vi "reportTaskState.vi"(7 "TaskRef":refnum<vi>, 8 "error in (no error)":errorcluster, 10 "Request":string, 11 "pdbm_taskroute_feedback_event":refnum<user-event>) -> (0 "error out":errorcluster, 3 "pdbm_taskroute_feedback_event out":refnum<user-event>, 5 "TaskRef out":refnum<vi>)   [LabVIEW 2015, in "pdbm_tasks.lvlib"]
uses:
  pdbm_tasks.lvlib
  pdbm_test_route/UsrDefine/TaskFeedbackCmd.ctl
  UsrDefine/TaskRequest.ctl
  pdbm_test_route/pdbm_task_route.lvlib
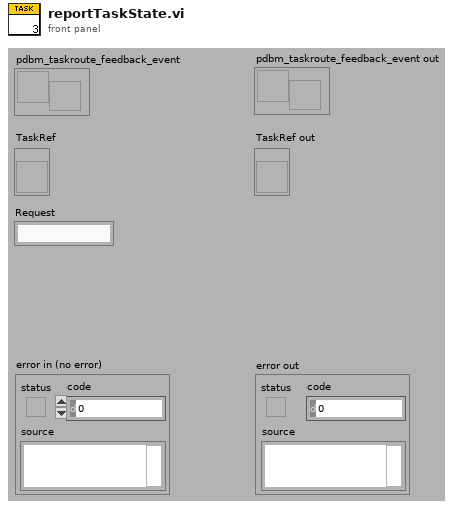
[diagram p1: front panel]
types:
  T1 = typedef "pdbm_tasks.lvlib/TaskRequest.ctl" = cluster{"Command":string, "Variant":variant}
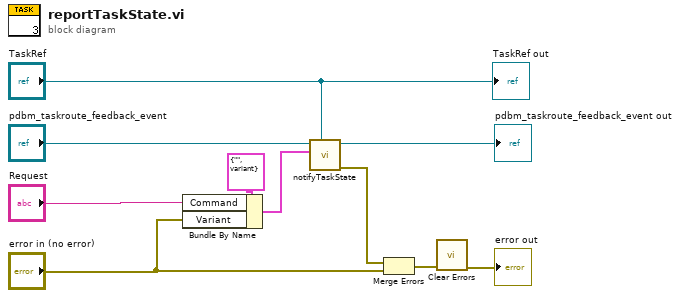
[diagram p0: block diagram]
diagram:
  n1 = Bundle By Name(cluster=T1 {"Command"="", "Variant"=variant} ("TaskRequest"), "Command"="Request", "Variant"="error in (no error)") -> (w7:T1)
  n2 = call "notifyTaskState.vi"("TaskRef"="TaskRef", "TaskRequest"=w7, "pdbm_taskroute_feedback_event"="pdbm_taskroute_feedback_event") -> ("error IO"=w3:errorcluster, "pdbm_taskroute_feedback_event out"=→"pdbm_taskroute_feedback_event out":refnum<user-event>)  [unwired: 7 in]
  n3 = Merge Errors(w3, "error in (no error)") -> (w2:errorcluster)
  n4 = call <vilib>:"Clear Errors.vi"("error in (no error)"=w2) -> ("error out"=→"error out":errorcluster)  [unwired: 5 in, 1 out]
  "TaskRef out" <- "TaskRef"
